vi "Stop Core.vi"(10 "final error code":i32, 11 "TestFixPtProc in":refnum<class "TestFixPtProc.lvclass">) -> (3 "TestFixPtProc out":refnum<class "TestFixPtProc.lvclass">)   [LabVIEW 2024, in "TestFixPtActor.lvlib" / "TestFixPtProc.lvclass"]
doc: "(<B>Filename</B>: Actor Framework.lvlib:Actor.lvclass:Stop Core.vi)\n\nDefines what the actor does before it stops. Use the <B>final error code</B> input to determine whether the actor shut down in response to an error.\n\nBy default, this method does nothing. A descendant class may override it to define behavior, such as shutting down any processes the actor initiated in its override of the Actor Core method."
uses:
  TestFixPtProc.lvclass
  TestFixPtProc.lvclass/TestFixPtProc.ctl
  <vilib>/ActorFramework/Actor/Actor.lvclass
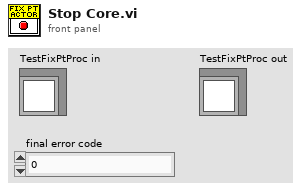
[diagram p1: front panel]
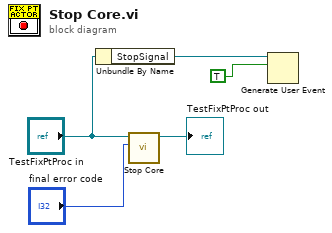
[diagram p0: block diagram]
diagram:
  n1 = Unbundle By Name("TestFixPtProc in") -> ("StopSignal"=w2:refnum<user-event>)
  n2 = call-parent "Stop Core.vi"("final error code"="final error code", "Actor in"="TestFixPtProc in") -> ("Actor out"=→"TestFixPtProc out":refnum<class "TestFixPtProc.lvclass">)  [unwired: 9 in]
  n3 = Generate User Event(user event=w2, event data cluster=TRUE) -> ()  [unwired: 2 in, 2 out]
